vi "Track(topview).vi"() -> ()   [LabVIEW 2014]
uses:
  <vilib>/Utility/file.llb/Write To Spreadsheet File (string).vi
  <vilib>/vision/NI_Vision_Development_Module.lvlib
panel:
  in  "Pause Button":bool
  out "Numeric":dbl
  in  "Start":bool
  in  "Stop Button":bool
  in  "Frame jump":i32=3
  out "Data":dbl[][](array[numeric])
  in  "Grab":bool
  out "Top VIew":cluster{"Numeric":dbl, "Numeric":dbl}[](graph)
  in  "Playback speed":u32(slide)=200
  in  "Progress":i32(slide) step=219843704 scale=-1.0..377.0
  in  "Video path":path
  out "Track":T1(plugin-control)
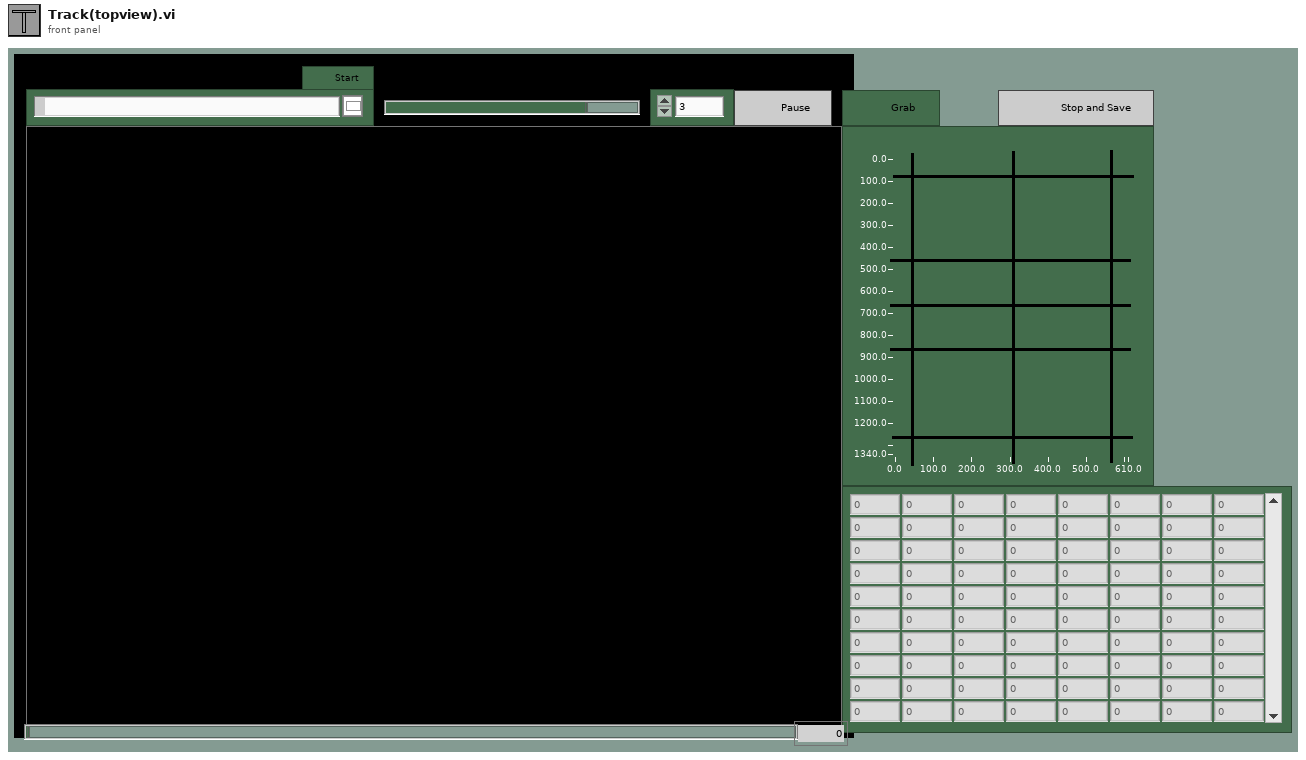
[diagram p1: front panel]
types:
  T1 = typedef "IMAQ Image.ctl" = refnum<image>
  T2 = typedef "Image Type" = u32
  T3 = typedef "AviRefnum.ctl" = refnum<k1>
  T4 = cluster{"width":u32, "height":u32, "framesPerSecond":u32, "compressionFilter":string, "hasData":bool}
  T5 = cluster{cluster{"X":sgl, "Y":sgl}[], cluster{i32, i32}[], "Unit":u32}
  T6 = cluster{"Origin Pixel":cluster{"X":sgl, "Y":sgl}, "Angle Relative to Horizontal (deg)":sgl, "Axis Reference":u32}
  T7 = typedef "Particle Parameters" = i32
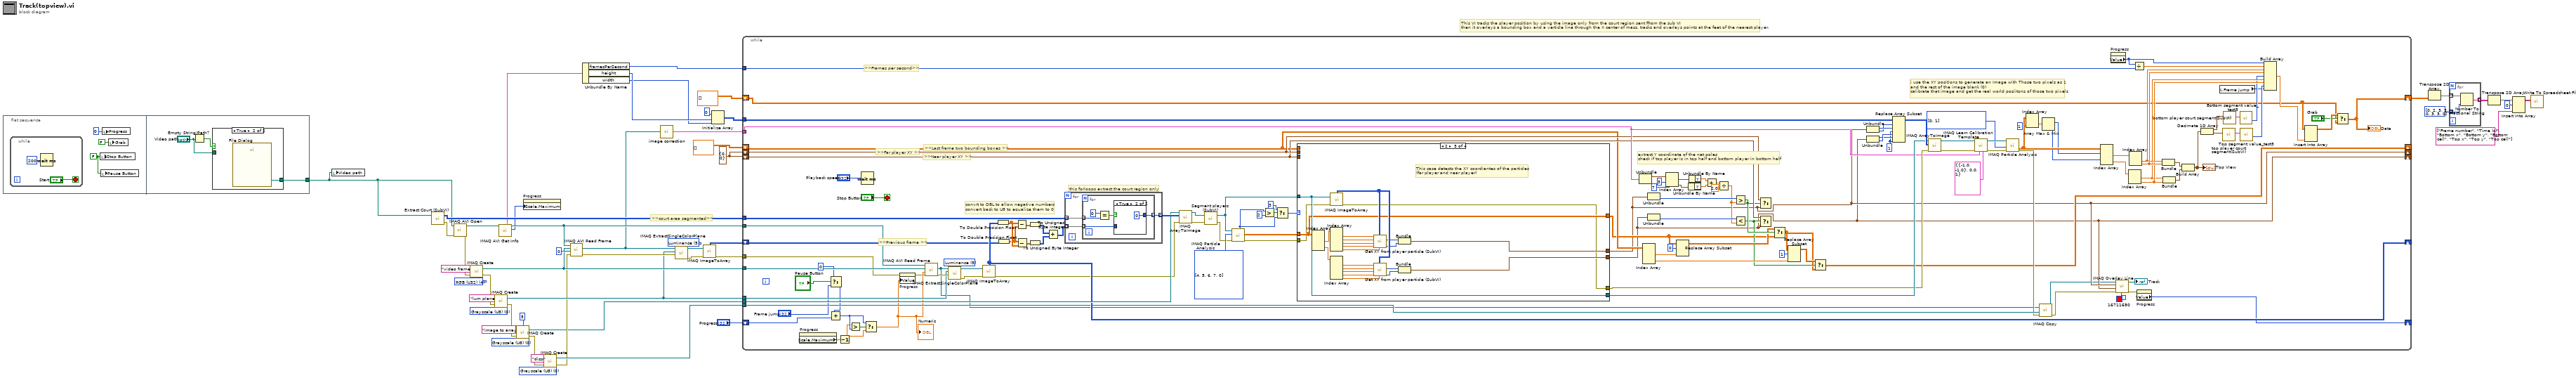
[diagram p0: block diagram]
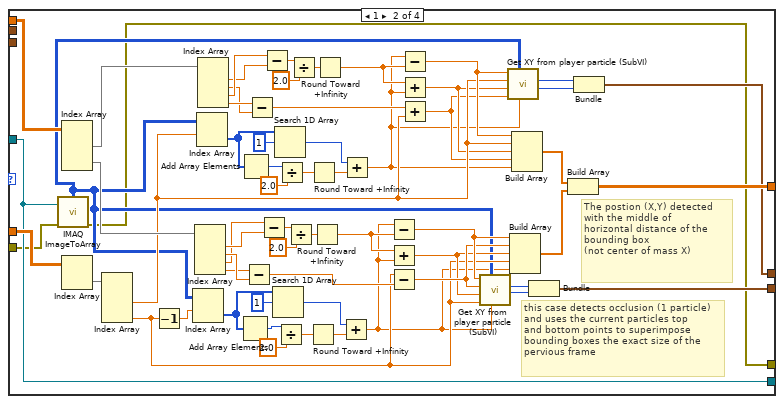
[diagram p4: hidden frame]
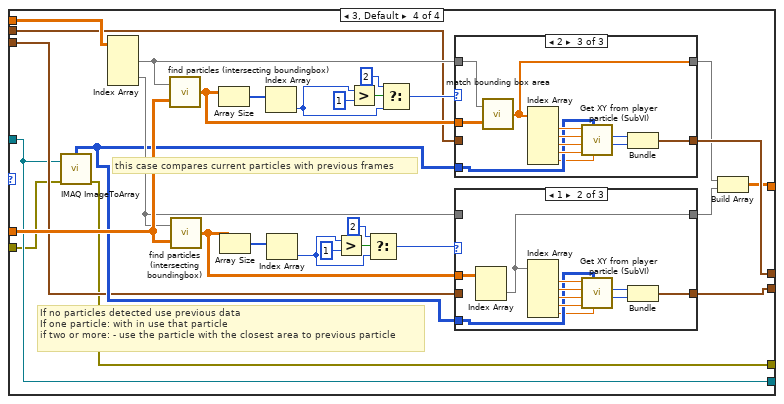
[diagram p5: hidden frame]
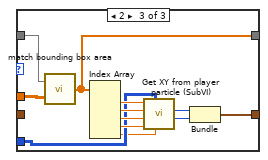
[diagram p7: hidden frame]
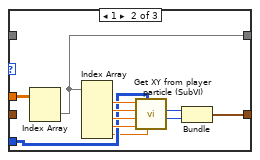
[diagram p9: hidden frame]
diagram:
  w24 = cluster{"X coordinate":i32, "Y coordinate":i32} {"X coordinate"=0, "Y coordinate"=0}
  w37 = T2 0 items=["Grayscale (U8)", "Grayscale (I16)", "Grayscale (SGL)", "Complex (CSG)", "RGB (U32)", "HSL (U32)", "RGB (U64)", "Grayscale (U16)"] ("Image Type")
  w44 = 5 items=["Red", "Green", "Blue", "Hue", "Saturation", "Luminance", "Value", "Intensity"] ("Color Plane")
  w45 = T2 0 items=["Grayscale (U8)", "Grayscale (I16)", "Grayscale (SGL)", "Complex (CSG)", "RGB (U32)", "HSL (U32)", "RGB (U64)", "Grayscale (U16)"] ("Image Type")
  w49 = T2 0 items=["Grayscale (U8)", "Grayscale (I16)", "Grayscale (SGL)", "Complex (CSG)", "RGB (U32)", "HSL (U32)", "RGB (U64)", "Grayscale (U16)"] ("Image Type")
  w47 = T2 4 items=["Grayscale (U8)", "Grayscale (I16)", "Grayscale (SGL)", "Complex (CSG)", "RGB (U32)", "HSL (U32)", "RGB (U64)", "Grayscale (U16)"] ("Image Type")
  # ">>court area segmented>>"
  # "This VI tracks the player position by using the image only from the court region sent ffrom the sub VI\nthen it overlays a bounding box and a verticle line through the X center of mass. tracks and overlays points at the feet of the nearest player."
  n1 = flat-sequence {
    tunnel: [w59] -> w3
    frame #0 {
      w52 = FALSE ("Stop Button")
      n2 = while {
        stop <- "Start" stop-if-true
        n3 = Wait (ms)(milliseconds to wait=u32 200) -> ()  [unwired: 1 out]
      }
      n4 = local write "Stop Button"(w52) -> ()
      n5 = local write "Pause Button"(w52) -> ()
      n6 = local write "Progress"(0 ("Progress")) -> ()
      n7 = local write "Grab"(FALSE ("Grab")) -> ()
    }
    frame #1 {
      n8 = Empty String/Path?(string/path="Video path") -> (empty?=w58:bool)
      n9 = case shown="True" w58 {
        tunnel: [w60 w61] -> w59
        tunnel: "Video path" -> [w60 _]
        frame False {
        }
        frame True {
          n10 = call "File Dialog"() -> ("selected path"=w61:path)  [unwired: 12 in, 3 out]
        }
      }
    }
  }
  n11 = local write "Video path"(w3) -> ()
  n12 = call "Extract Court (SubVI).vi"("AVI Path"=w3) -> ("error out"=w51:errorcluster, "Court pixels out"=w27:u8[][])  [unwired: 1 in]
  n13 = call "IMAQ AVI Open"("error in (no error)"=w51, "AVI Path"=w3) -> ("error out"=w33:errorcluster, "Avi Refnum"=w22:T3)  [unwired: 8 in]
  n14 = call "IMAQ Create"("Image Name"="video frame", "Image Type"=w47, "error in (no error)"=w33) -> ("New Image"=w41:T1, "error out"=w32:errorcluster)  [unwired: 2 in]
  n15 = call "IMAQ Create"("Image Name"="lum plane", "Image Type"=w49, "error in (no error)"=w32) -> ("New Image"=w40:T1, "error out"=w31:errorcluster)  [unwired: 2 in]
  n16 = call "IMAQ AVI Get Info"("Avi Refnum"=w22) -> ("Number of Frames"=w20:u32, "Avi Refnum (duplicate)"=w21:T3, "Frame Data"=w17:T4)  [unwired: 6 in, 2 out]
  n17 = call "IMAQ Create"("Border Size"=5, "Image Name"="image to array", "Image Type"=w45, "error in (no error)"=w31) -> ("New Image"=w26:T1, "error out"=w30:errorcluster)  [unwired: 1 in]
  n18 = property on="Progress" class="Slide (strict)"("Scale.Maximum"=w20) -> ()  [unwired: 2 in, 2 out]
  n19 = call "IMAQ Create"("Image Name"="disp", "Image Type"=w37, "error in (no error)"=w30) -> ("New Image"=w35:T1, "error out"=w29:errorcluster)  [unwired: 2 in]
  n20 = call "IMAQ AVI Read Frame"("error in (no error)"=w29, "Frame Number"=u32 0, "Image"=w41, "Avi Refnum"=w21) -> ("error out"=w43:errorcluster, "Image Out"=w1:T1)  [unwired: 4 in, 2 out]
  n21 = Unbundle By Name(w17) -> ("framesPerSecond"=w12:u32, "height"=w16:u32, "width"=w15:u32)
  n22 = call "image correction.vi"("Image"=w1) -> ("ref points"=w2:T5)
  n23 = call "IMAQ ExtractSingleColorPlane"("Color Plane"=w44, "error in (no error)"=w43, "Image Dst"=w40, "Image Src"=w1) -> ("error out"=w34:errorcluster, "Image Dst Out"=w38:T1)  [unwired: 6 in]
  n24 = call "IMAQ ImageToArray"("error in (no error)"=w34, "Image"=w38) -> ("error out"=w19:errorcluster, "Image Pixels (U8)"=w39:u8[][])  [unwired: 2 in, 3 out]
  n25 = Initialize Array(u8 0 ("element"), w16, w15) -> (w14:u8[][])
  n26 = while {
    tunnel: w21 -> [w155]
    tunnel: w41 -> [w171]
    tunnel: w27 -> [w187]
    tunnel: w40 -> [w172]
    tunnel: w26 -> [w185]
    shift-right: [w184] -> _
    shift-left: w39 -> [w183]
    tunnel: w35 -> [w157]
    shift-right: [w102] -> _
    shift-left: dbl[][] [] ("Particle Measurements (Pixels)") -> [w112]
    shift-right: [w100] -> _
    shift-left: w24 -> [w114]
    shift-right: [w99] -> _
    shift-left: w24 -> [w113]
    shift-right: [w151] -> _
    shift-left: "Progress" -> [w156]
    tunnel: w19 -> [w154]
    tunnel: w14 -> [w150]
    tunnel: w2 -> [w127]
    shift-right: [w128] -> w5
    shift-left: dbl[][] [] -> [w74]
    tunnel: w12 -> [w92]
    stop <- "Stop Button" stop-if-true
    w136 = T7[] [0, 1] items=["Center of Mass X", "Center of Mass Y", "First Pixel X", "First Pixel Y", "Bounding Rect Left", "Bounding Rect Top", "Bounding Rect Right", "Bounding Rect Bottom", "Max Feret Diameter Start X", "Max Feret Diameter Start Y", "Max Feret Diameter End X", "Max Feret Diameter End Y", "Max Horiz. Segment Length Left", "Max Horiz. Segment Length Right", "Max Horiz. Segment Length Row", "-", "Bounding Rect Width", "Bounding Rect Height", "Bounding Rect Diagonal", "Perimeter", "Convex Hull Perimeter", "Holes' Perimeter", "Max Feret Diameter", "Equivalent Ellipse Major Axis", "Equivalent Ellipse Minor Axis", "Equivalent Ellipse Minor Axis (Feret)", "Equivalent Rect Long Side", "Equivalent Rect Short Side", "Equivalent Rect Diagonal", "Equivalent Rect Short Side (Feret)", "Average Horiz. Segment Length", "Average Vert. Segment Length", "Hydraulic Radius", "Waddel Disk Diameter", "-", "Area", "Holes' Area", "Particle & Holes' Area", "Convex Hull Area", "Image Area", "-", "Number of Holes", "Number of Horiz. Segments", "Number of Vert. Segments", "-", "Orientation", "Max Feret Diameter Orientation", "-", "% Area/Image Area", "% Area/(Particle & Holes' Area)", "Ratio of Equivalent Ellipse Axes", "Ratio of Equivalent Rect Sides", "-", "Elongation Factor", "Compactness Factor", "Heywood Circularity Factor", "Type Factor", "-", "Sum X", "Sum Y", "Sum XX", "Sum XY", "Sum YY", "Sum XXX", "Sum XXY", "Sum XYY", "Sum YYY", "-", "Moment of Inertia XX", "Moment of Inertia XY", "Moment of Inertia YY", "Moment of Inertia XXX", "Moment of Inertia XXY", "Moment of Inertia XYY", "Moment of Inertia YYY", "Norm. Moment of Inertia XX", "Norm. Moment of Inertia XY", "Norm. Moment of Inertia YY", "Norm. Moment of Inertia XXX", "Norm. Moment of Inertia XXY", "Norm. Moment of Inertia XYY", "Norm. Moment of Inertia YYY", "Hu Moment 1", "Hu Moment 2", "Hu Moment 3", "Hu Moment 4", "Hu Moment 5", "Hu Moment 6", "Hu Moment 7"] ("Real-World Measurements")
    w145 = u8 1 ("new element/subarray")
    w173 = T7[] [4, 5, 6, 7, 0] items=["Center of Mass X", "Center of Mass Y", "First Pixel X", "First Pixel Y", "Bounding Rect Left", "Bounding Rect Top", "Bounding Rect Right", "Bounding Rect Bottom", "Max Feret Diameter Start X", "Max Feret Diameter Start Y", "Max Feret Diameter End X", "Max Feret Diameter End Y", "Max Horiz. Segment Length Left", "Max Horiz. Segment Length Right", "Max Horiz. Segment Length Row", "-", "Bounding Rect Width", "Bounding Rect Height", "Bounding Rect Diagonal", "Perimeter", "Convex Hull Perimeter", "Holes' Perimeter", "Max Feret Diameter", "Equivalent Ellipse Major Axis", "Equivalent Ellipse Minor Axis", "Equivalent Ellipse Minor Axis (Feret)", "Equivalent Rect Long Side", "Equivalent Rect Short Side", "Equivalent Rect Diagonal", "Equivalent Rect Short Side (Feret)", "Average Horiz. Segment Length", "Average Vert. Segment Length", "Hydraulic Radius", "Waddel Disk Diameter", "-", "Area", "Holes' Area", "Particle & Holes' Area", "Convex Hull Area", "Image Area", "-", "Number of Holes", "Number of Horiz. Segments", "Number of Vert. Segments", "-", "Orientation", "Max Feret Diameter Orientation", "-", "% Area/Image Area", "% Area/(Particle & Holes' Area)", "Ratio of Equivalent Ellipse Axes", "Ratio of Equivalent Rect Sides", "-", "Elongation Factor", "Compactness Factor", "Heywood Circularity Factor", "Type Factor", "-", "Sum X", "Sum Y", "Sum XX", "Sum XY", "Sum YY", "Sum XXX", "Sum XXY", "Sum XYY", "Sum YYY", "-", "Moment of Inertia XX", "Moment of Inertia XY", "Moment of Inertia YY", "Moment of Inertia XXX", "Moment of Inertia XXY", "Moment of Inertia XYY", "Moment of Inertia YYY", "Norm. Moment of Inertia XX", "Norm. Moment of Inertia XY", "Norm. Moment of Inertia YY", "Norm. Moment of Inertia XXX", "Norm. Moment of Inertia XXY", "Norm. Moment of Inertia XYY", "Norm. Moment of Inertia YYY", "Hu Moment 1", "Hu Moment 2", "Hu Moment 3", "Hu Moment 4", "Hu Moment 5", "Hu Moment 6", "Hu Moment 7"] ("Pixel Measurements")
    w188 = 5 items=["Red", "Green", "Blue", "Hue", "Saturation", "Luminance", "Value", "Intensity"] ("Color Plane")
    # ">>Frames per second>>"
    # "extract Y coordinate of the net poles\ncheck if top player is in top half and bottom player in bottom half"
    # "i use the XY positions to generate an Image with Those two pixels as 1 \nand the rest of the image blank (0)\ncalibrate that image and get the real world posiitons of those two pixels"
    # ">>Last frame two bounding boxes >>"
    # ">>Far player XY >>"
    # ">>Near player XY >>"
    # ">>Previous frame >>"
    # "convrt to DBL to allow negative numbers\nconvert back to U8 to equalize them to 0"
    # "this forloops extract the court region only"
    n27 = property on="Progress" class="Slide (strict)"() -> ("Scale.Maximum"=w72:dbl)  [unwired: 2 in, 2 out]
    n28 = Select(t=0, s="Pause Button", f="Frame jump") -> (s? t:f=w64:i32)
    n29 = Add(x=w64, y=w156) -> (x+y=w70:i32)
    n30 = Decrement(x=w72) -> (x-1=w69:dbl)
    n31 = Greater?(x=w69, y=w70) -> (0:w71:bool)
    n32 = Wait (ms)(milliseconds to wait="Playback speed") -> ()  [unwired: 1 out]
    n33 = Select(t=w70, s=w71, f=w69) -> (s? t:f=w62:dbl)
    "Numeric" <- w62
    n34 = property on="Progress" class="Slide (strict)"(error in=w154, "Value"=w62) -> (error out=w153:errorcluster)  [unwired: 1 in, 1 out]
    n35 = call "IMAQ AVI Read Frame"("error in (no error)"=w153, "Frame Number"=w62, "Image"=w171, "Avi Refnum"=w155) -> ("error out"=w189:errorcluster, "Image Out"=w90:T1)  [unwired: 4 in, 2 out]
    n36 = call "IMAQ ExtractSingleColorPlane"("Color Plane"=w188, "error in (no error)"=w189, "Image Dst"=w172, "Image Src"=w90) -> ("error out"=w175:errorcluster, "Image Dst Out"=w89:T1)  [unwired: 6 in]
    n37 = call "IMAQ ImageToArray"("error in (no error)"=w175, "Image"=w89) -> ("error out"=w174:errorcluster, "Image Pixels (U8)"=w184:u8[][])  [unwired: 2 in, 3 out]
    n38 = To Double Precision Float(number=w184) -> (double precision float=w179:dbl[][])
    n39 = To Double Precision Float(number=w183) -> (double precision float=w178:dbl[][])
    n40 = Subtract(x=w179, y=w178) -> (x-y=w177:dbl[][])
    n41 = Subtract(x=w178, y=w179) -> (x-y=w176:dbl[][])
    n42 = To Unsigned Byte Integer(number=w177) -> (unsigned 8bit integer=w182:u8[][])
    n43 = To Unsigned Byte Integer(number=w176) -> (unsigned 8bit integer=w181:u8[][])
    n44 = Add(x=w182, y=w181) -> (x+y=w180:u8[][])
    n45 = for {
      tunnel: w187 -> [w360] mode=indexing
      tunnel: [w359] -> w186 mode=indexing
      tunnel: w180 -> [w358] mode=indexing
      n46 = for {
        tunnel: w360 -> [w365] mode=indexing
        tunnel: [w362] -> w359 mode=indexing
        tunnel: w358 -> [w361] mode=indexing
        n47 = Equal?(x=u8 0, y=w365) -> (x = y?=w363:bool)
        n48 = case shown="True" w363 {
          tunnel: [w366 u8 0 ("x")] -> w362
          tunnel: w361 -> [w366 _]
          frame False {
          }
          frame True {
          }
        }
      }
    }
    n49 = call "IMAQ ArrayToImage"("error in (no error)"=w174, "Image Pixels (U8)"=w186, "Image"=w185) -> ("error out"=w169:errorcluster, "Image Out"=w170:T1)  [unwired: 7 in]
    n50 = call "Segment players (SubVI).vi"("error In"=w169, "Image In"=w170) -> ("error out"=w163:errorcluster, "Image Out"=w161:T1)
    n51 = call "IMAQ Particle Analysis"("error in (no error)"=w163, "Pixel Measurements"=w173, "Image"=w161) -> ("error out"=w162:errorcluster, "Particle Measurements (Pixels)"=w160:dbl[][], "Number of Particles"=w165:i32)  [unwired: 3 in, 3 out]
    n52 = Greater?(x=w165, y=2) -> (0:w168:bool)
    n53 = Select(t=3 ("y"), s=w168, f=w165) -> (s? t:f=w164:i32)
    n54 = case shown="2" w164 {
      tunnel: [w193 w220 w274 w284] -> w143
      tunnel: w160 -> [_ w255 w262 w304]
      tunnel: w162 -> [w190 w196 w259 w280]
      tunnel: w161 -> [w193 w220 w274 w284]
      tunnel: [w191 w204 w264 w286] -> w99
      tunnel: [w192 w211 w263 w285] -> w100
      tunnel: [w194 w221 w262 w281] -> w101
      tunnel: w112 -> [w194 w245 _ w307]
      tunnel: w114 -> [w192 _ _ w292]
      tunnel: w113 -> [w191 _ _ w287]
      tunnel: [w190 w195 w258 w279] -> w142
      frame 0 {
        # "This case identifies frames where no particles are detected and keeps the same values from the\nprevious frame"
      }
      frame 1 {
        # "The postion (X,Y) detected with the middle of \nhorizontal distance of the bounding box\n(not center of mass X)"
        # "this case detects occlusion (1 particle)\nand uses the current particles top \nand bottom points to superimpose \nbounding boxes the exact size of the \npervious frame"
        n55 = call "IMAQ ImageToArray"("error in (no error)"=w196, "Image"=w220) -> ("error out"=w195:errorcluster, "Image Pixels (U8)"=w203:u8[][])  [unwired: 2 in, 3 out]
        n56 = Index Array(array=w245) -> (element #1=w253:dbl[], element #2=w225:dbl[])  [unwired: 4 in]
        n57 = Index Array(array=w255) -> (element=w254:dbl[])  [unwired: 2 in]
        n58 = Index Array(array=w254) -> (element #2=w216:dbl, element #4=w207:dbl)  [unwired: 4 in, 2 out]
        n59 = Decrement(x=w207) -> (x-1=w218:dbl)
        n60 = Index Array(array=w203, index (row)=w218) -> (element=w240:u8[])  [unwired: 1 in]
        n61 = Index Array(array=w225) -> (element #1=w229:dbl, element #2=w232:dbl, element #3=w228:dbl, element #4=w231:dbl)  [unwired: 4 in]
        n62 = Index Array(array=w203, index (row)=w216) -> (element=w233:u8[])  [unwired: 1 in]
        n63 = Index Array(array=w253) -> (element #1=w249:dbl, element #2=w246:dbl, element #3=w250:dbl, element #4=w247:dbl)  [unwired: 4 in]
        n64 = Add Array Elements(numeric array=w240) -> (sum=w241:u8)
        n65 = Add Array Elements(numeric array=w233) -> (sum=w237:u8)
        n66 = Subtract(x=w231, y=w232) -> (x-y=w219:dbl)
        n67 = Subtract(x=w247, y=w246) -> (x-y=w224:dbl)
        n68 = Subtract(x=w228, y=w229) -> (x-y=w227:dbl)
        n69 = Subtract(x=w250, y=w249) -> (x-y=w251:dbl)
        n70 = Search 1D Array(1D array=w240, element=u8 1) -> (index of element=w239:i32)  [unwired: 1 in]
        n71 = Search 1D Array(1D array=w233, element=u8 1) -> (index of element=w238:i32)  [unwired: 1 in]
        n72 = Divide(x=w241, y=2.0) -> (x/y=w242:dbl)
        n73 = Divide(x=w237, y=2.0) -> (x/y=w236:dbl)
        n74 = Divide(x=w227, y=2.0) -> (x/y=w230:dbl)
        n75 = Divide(x=w251, y=2.0) -> (x/y=w248:dbl)
        n76 = Round Toward +Infinity(x=w242) -> (ceil(x): smallest int >= x=w201:dbl)
        n77 = Round Toward +Infinity(x=w236) -> (ceil(x): smallest int >= x=w200:dbl)
        n78 = Round Toward +Infinity(x=w230) -> (ceil(x): smallest int >= x=w202:dbl)
        n79 = Round Toward +Infinity(x=w248) -> (ceil(x): smallest int >= x=w199:dbl)
        n80 = Add(x=w239, y=w201) -> (x+y=w197:dbl)
        n81 = Add(x=w238, y=w200) -> (x+y=w198:dbl)
        n82 = Subtract(x=w197, y=w202) -> (x-y=w210:dbl)
        n83 = Add(x=w202, y=w197) -> (x+y=w208:dbl)
        n84 = Subtract(x=w207, y=w219) -> (x-y=w209:dbl)
        n85 = Subtract(x=w198, y=w199) -> (x-y=w217:dbl)
        n86 = Add(x=w199, y=w198) -> (x+y=w215:dbl)
        n87 = Add(x=w224, y=w216) -> (x+y=w214:dbl)
        n88 = call "Get XY from player particle (SubVI).vi"("Center of mass X"=w197, "Image in Pixels (U8)"=w203, "Particle bounding rect bottom"=w207, "Particle bounding rect right"=w208, "Particle bounding rect top"=w209, "Particle bounding rect left"=w210) -> ("Y coordinate"=w205:i32, "X coordinate"=w206:i32)  [unwired: 1 in, 1 out]
        n89 = call "Get XY from player particle (SubVI).vi"("Center of mass X"=w198, "Image in Pixels (U8)"=w203, "Particle bounding rect bottom"=w214, "Particle bounding rect right"=w215, "Particle bounding rect top"=w216, "Particle bounding rect left"=w217) -> ("Y coordinate"=w212:i32, "X coordinate"=w213:i32)  [unwired: 1 in, 1 out]
        n90 = Build Array(w210, w209, w208, w207, w197) -> (w222:dbl[])
        n91 = Build Array(w217, w216, w215, w214, w198) -> (w223:dbl[])
        n92 = Bundle("X coordinate"=w206, "Y coordinate"=w205) -> (w204:cluster{"X coordinate":i32, "Y coordinate":i32})  [unwired: 1 in]
        n93 = Build Array(w223, w222) -> (w221:dbl[][])
        n94 = Bundle("X coordinate"=w213, "Y coordinate"=w212) -> (w211:cluster{"X coordinate":i32, "Y coordinate":i32})  [unwired: 1 in]
      }
      frame 2 {
        # "This case detects the XY coordiantes of the particles\n(far player and near player)"
        n95 = Index Array(array=w262) -> (element #1=w268:dbl[], element #2=w267:dbl[])  [unwired: 4 in]
        n96 = call "IMAQ ImageToArray"("error in (no error)"=w259, "Image"=w274) -> ("error out"=w258:errorcluster, "Image Pixels (U8)"=w269:u8[][])  [unwired: 2 in, 3 out]
        n97 = Index Array(array=w268) -> (element #1=w278:dbl, element #2=w277:dbl, element #3=w276:dbl, element #4=w275:dbl, element #5=w261:dbl)  [unwired: 5 in]
        n98 = Index Array(array=w267) -> (element #1=w270:dbl, element #2=w271:dbl, element #3=w272:dbl, element #4=w273:dbl, element #5=w260:dbl)  [unwired: 5 in]
        n99 = call "Get XY from player particle (SubVI).vi"("Center of mass X"=w261, "Image in Pixels (U8)"=w269, "Particle bounding rect bottom"=w275, "Particle bounding rect right"=w276, "Particle bounding rect top"=w277, "Particle bounding rect left"=w278) -> ("Y COM"=w257:i32, "X coordinate"=w266:i32)  [unwired: 1 in, 1 out]
        n100 = call "Get XY from player particle (SubVI).vi"("Center of mass X"=w260, "Image in Pixels (U8)"=w269, "Particle bounding rect bottom"=w273, "Particle bounding rect right"=w272, "Particle bounding rect top"=w271, "Particle bounding rect left"=w270) -> ("Y COM"=w256:i32, "X coordinate"=w265:i32)  [unwired: 1 in, 1 out]
        n101 = Bundle("X coordinate"=w266, "Y COM"=w257) -> (w263:cluster{"X coordinate":i32, "Y COM":i32})  [unwired: 1 in]
        n102 = Bundle("X coordinate"=w265, "Y COM"=w256) -> (w264:cluster{"X coordinate":i32, "Y COM":i32})  [unwired: 1 in]
      }
      frame 3, Default {
        # "If no particles detected use previous data\nIf one particle: with in use that particle\nif two or more: - use the particle with the closest area to previous particle"
        # "this case compares current particles with previous frames"
        n103 = call "IMAQ ImageToArray"("error in (no error)"=w280, "Image"=w284) -> ("error out"=w279:errorcluster, "Image Pixels (U8)"=w288:u8[][])  [unwired: 2 in, 3 out]
        n104 = Index Array(array=w307) -> (element #1=w303:dbl[], element #2=w291:dbl[])  [unwired: 4 in]
        n105 = call "find particles (intersecting boundingbox).vi"("Particle Measurements in (bounding boxes)"=w304, "bounding box in"=w303) -> ("Particles within bounding box"=w302:dbl[][])
        n106 = call "find particles (intersecting boundingbox).vi"("Particle Measurements in (bounding boxes)"=w304, "bounding box in"=w291) -> ("Particles within bounding box"=w289:dbl[][])
        n107 = Array Size(array=w302) -> (size(s)=w306:i32[])
        n108 = Array Size(array=w289) -> (size(s)=w305:i32[])
        n109 = Index Array(array=w306) -> (element=w294:i32)  [unwired: 1 in]
        n110 = Index Array(array=w305) -> (element=w295:i32)  [unwired: 1 in]
        n111 = Greater?(x=w295, y=1) -> (0:w298:bool)
        n112 = Greater?(x=w294, y=1) -> (0:w299:bool)
        n113 = Select(t=2 ("y"), s=w298, f=w295) -> (s? t:f=w290:i32)
        n114 = Select(t=2 ("y"), s=w299, f=w294) -> (s? t:f=w293:i32)
        n115 = case shown="2" w293 {
          tunnel: w303 -> [w334 _ w349]
          tunnel: w302 -> [_ w345 w348]
          tunnel: [w334 w336 w347] -> w283
          tunnel: w288 -> [_ w338 w351]
          tunnel: [w333 w337 w350] -> w285
          tunnel: w292 -> [w333 _ _]
          frame 0, Default {
          }
          frame 1 {
            n116 = Index Array(array=w345) -> (element=w336:dbl[])  [unwired: 2 in]
            n117 = Index Array(array=w336) -> (element #1=w342:dbl, element #2=w341:dbl, element #3=w340:dbl, element #4=w339:dbl, element #5=w335:dbl)  [unwired: 5 in]
            n118 = call "Get XY from player particle (SubVI).vi"("Center of mass X"=w335, "Image in Pixels (U8)"=w338, "Particle bounding rect bottom"=w339, "Particle bounding rect right"=w340, "Particle bounding rect top"=w341, "Particle bounding rect left"=w342) -> ("Y coordinate"=w343:i32, "X coordinate"=w344:i32)  [unwired: 1 in, 1 out]
            n119 = Bundle("X coordinate"=w344, "Y coordinate"=w343) -> (w337:cluster{"X coordinate":i32, "Y coordinate":i32})  [unwired: 1 in]
          }
          frame 2 {
            n120 = call "match bounding box area.vi"("particle measurements (bounding box)"=w348, "bounding box in"=w349) -> ("matching bounding box"=w347:dbl[])
            n121 = Index Array(array=w347) -> (element #1=w355:dbl, element #2=w354:dbl, element #3=w353:dbl, element #4=w352:dbl, element #5=w346:dbl)  [unwired: 5 in]
            n122 = call "Get XY from player particle (SubVI).vi"("Center of mass X"=w346, "Image in Pixels (U8)"=w351, "Particle bounding rect bottom"=w352, "Particle bounding rect right"=w353, "Particle bounding rect top"=w354, "Particle bounding rect left"=w355) -> ("Y coordinate"=w356:i32, "X coordinate"=w357:i32)  [unwired: 1 in, 1 out]
            n123 = Bundle("X coordinate"=w357, "Y coordinate"=w356) -> (w350:cluster{"X coordinate":i32, "Y coordinate":i32})  [unwired: 1 in]
          }
        }
        n124 = case shown="1" w290 {
          tunnel: w291 -> [w309 _ w324]
          tunnel: w289 -> [_ w320 w323]
          tunnel: [w309 w311 w322] -> w282
          tunnel: w288 -> [_ w313 w326]
          tunnel: [w308 w312 w325] -> w286
          tunnel: w287 -> [w308 _ _]
          frame 0, Default {
          }
          frame 1 {
            n125 = Index Array(array=w320) -> (element=w311:dbl[])  [unwired: 2 in]
            n126 = Index Array(array=w311) -> (element #1=w317:dbl, element #2=w316:dbl, element #3=w315:dbl, element #4=w314:dbl, element #5=w310:dbl)  [unwired: 5 in]
            n127 = call "Get XY from player particle (SubVI).vi"("Center of mass X"=w310, "Image in Pixels (U8)"=w313, "Particle bounding rect bottom"=w314, "Particle bounding rect right"=w315, "Particle bounding rect top"=w316, "Particle bounding rect left"=w317) -> ("Y coordinate"=w318:i32, "X coordinate"=w319:i32)  [unwired: 1 in, 1 out]
            n128 = Bundle("X coordinate"=w319, "Y coordinate"=w318) -> (w312:cluster{"X coordinate":i32, "Y coordinate":i32})  [unwired: 1 in]
          }
          frame 2 {
            n129 = call "match bounding box area.vi"("particle measurements (bounding box)"=w323, "bounding box in"=w324) -> ("matching bounding box"=w322:dbl[])
            n130 = Index Array(array=w322) -> (element #1=w330:dbl, element #2=w329:dbl, element #3=w328:dbl, element #4=w327:dbl, element #5=w321:dbl)  [unwired: 5 in]
            n131 = call "Get XY from player particle (SubVI).vi"("Center of mass X"=w321, "Image in Pixels (U8)"=w326, "Particle bounding rect bottom"=w327, "Particle bounding rect right"=w328, "Particle bounding rect top"=w329, "Particle bounding rect left"=w330) -> ("Y coordinate"=w331:i32, "X coordinate"=w332:i32)  [unwired: 1 in, 1 out]
            n132 = Bundle("X coordinate"=w332, "Y coordinate"=w331) -> (w325:cluster{"X coordinate":i32, "Y coordinate":i32})  [unwired: 1 in]
          }
        }
        n133 = Build Array(w283, w282) -> (w281:dbl[][])
      }
    }
    n134 = Unbundle(w127) -> (w126:cluster{"X":sgl, "Y":sgl}[])  [unwired: 2 out]
    n135 = Index Array(array=w112) -> (element #1=w110:dbl[], element #2=w106:dbl[])  [unwired: 4 in]
    n136 = Unbundle(w99) -> ("Y coordinate"=w116:i32)  [unwired: 1 out]
    n137 = Unbundle(w100) -> ("Y coordinate"=w117:i32)  [unwired: 1 out]
    n138 = Index Array(array=w126, index #1=3 ("index"), index #2=7 ("index")) -> (element #1=w123:cluster{"X":sgl, "Y":sgl}, element #2=w122:cluster{"X":sgl, "Y":sgl})
    n139 = Replace Array Subset(array=w101, new element=w110, index (row)=0) -> (w109:dbl[][])  [unwired: 1 in]
    n140 = Unbundle By Name(w122) -> ("Y"=w120:sgl)
    n141 = Unbundle By Name(w123) -> ("Y"=w121:sgl)
    n142 = Add(x=w121, y=w120) -> (x+y=w119:sgl)
    n143 = Divide(x=w119, y=sgl 2.0) -> (x/y=w115:sgl)
    n144 = Greater?(x=w117, y=w115) -> (0:w111:bool)
    n145 = Less?(x=w116, y=w115) -> (x < y?=w104:bool)
    n146 = Select(t=w114, s=w111, f=w100) -> ()  [unwired: 1 out]
    n147 = Select(t=w113, s=w104, f=w99) -> ()  [unwired: 1 out]
    n148 = Select(t=w109, s=w111, f=w101) -> (s? t:f=w103:dbl[][])
    n149 = Replace Array Subset(array=w103, new element=w106, index (row)=1) -> (w105:dbl[][])  [unwired: 1 in]
    n150 = Select(t=w105, s=w104, f=w103) -> (s? t:f=w102:dbl[][])
    n151 = Unbundle(w99) -> ("X coordinate"=w146:i32, "Y coordinate"=w147:i32)
    n152 = Unbundle(w100) -> ("X coordinate"=w149:i32, "Y coordinate"=w148:i32)
    n153 = Replace Array Subset(array=w150, new element #1=w145, index (row) #1=w148, index (col) #1=w149, new element #2=w145, index (row) #2=w147, index (col) #2=w146) -> (w144:u8[][])
    n154 = call "IMAQ ArrayToImage"("error in (no error)"=w142, "Image Pixels (U8)"=w144, "Image"=w143) -> ("error out"=w139:errorcluster, "Image Out"=w140:T1)  [unwired: 7 in]
    n155 = call "IMAQ Learn Calibration Template"("Calibration Axis Info"=T6 {"Origin Pixel"={"X"=-1.0, "Y"=-1.0}, "Angle Relative to Horizontal (deg)"=0.0, "Axis Reference"=1}, "Reference Points"=w127, "error in (no error)"=w139, "Image"=w140) -> ("error out"=w138:errorcluster, "Calibrated Image"=w137:T1)  [unwired: 5 in, 1 out]
    n156 = call "IMAQ Particle Analysis"("error in (no error)"=w138, "Real-World Measurements"=w136, "Image"=w137) -> ("error out"=w135:errorcluster, "Particle Measurements (Real-World)"=w85:dbl[][])  [unwired: 3 in, 4 out]
    n157 = Index Array(array=w85, index (col)=1 ("disabled index (col)")) -> (element=w83:dbl[])  [unwired: 1 in]
    n158 = call "IMAQ Copy"("error in (no error)"=w135, "Image Dst"=w157, "Image Src"=w90) -> ("error out"=w97:errorcluster, "Image Dst Out"=w98:T1)  [unwired: 3 in]
    n159 = Array Max & Min(array=w83) -> (max index (indices)=w82:i32, min index (indices)=w81:i32)  [unwired: 2 out]
    n160 = Index Array(array=w85, index (row) #1=w82, index (row) #2=w81) -> (element #1=w134:dbl[], element #2=w133:dbl[])  [unwired: 2 in]
    n161 = property on="Progress" class="Slide (strict)"() -> ("Value"=w93:i32)  [unwired: 2 in, 2 out]
    n162 = call "IMAQ Overlay Line"("Color"=u32 16711680, "error in (no error)"=w97, "End Point"=w99, "Start Point"=w100, "Image"=w98) -> ("error out"=w152:errorcluster, "Image Out"=→"Track":T1)  [unwired: 5 in]
    n163 = Index Array(array=w133) -> (element #1=w76:dbl, element #2=w77:dbl)  [unwired: 2 in]
    n164 = Index Array(array=w134) -> (element #1=w96:dbl, element #2=w95:dbl)  [unwired: 2 in]
    n165 = Divide(x=w93, y=w92) -> (x/y=w91:dbl)
    n166 = property on="Progress" class="Slide (strict)"(error in=w152) -> ("Value"=w151:i32)  [unwired: 1 in, 2 out]
    n167 = Bundle("Numeric"=w96, "Numeric"=w95) -> (w130:cluster{"Numeric":dbl, "Numeric":dbl})  [unwired: 1 in]
    n168 = Bundle("Numeric"=w76, "Numeric"=w77) -> (w129:cluster{"Numeric":dbl, "Numeric":dbl})  [unwired: 1 in]
    n169 = Build Array(w130, w129) -> (w88:cluster{"Numeric":dbl, "Numeric":dbl}[])
    "Top VIew" <- w88
    n170 = Decimate 1D Array(w88) -> (w80:cluster{"Numeric":dbl, "Numeric":dbl}[], w79:cluster{"Numeric":dbl, "Numeric":dbl}[])
    n171 = local read "Frame jump"() -> (w68:i32)
    n172 = call "top player court segment(SubVI).vi"("Top player position"=w79) -> ("Top player segment position"=w87:string)  [unwired: 10 in]
    n173 = call "bottom player court segment(SubVI).vi"("Bottom player position"=w80) -> ("Bottom player segment position"=w86:string)  [unwired: 10 in]
    n174 = call "Bottom segment value_test3.vi"("Bottom player segment position"=w86) -> ("Bottom player segment"=w75:i32)  [unwired: 9 in, 1 out]
    n175 = call "Top segment value_test3.vi"("Top player segment position"=w87) -> ("Top player segment value"=w78:i32)  [unwired: 9 in, 1 out]
    n176 = Build Array(w93, w91, w96, w95, w75, w76, w77, w78, w68) -> (w94:dbl[])
    n177 = Insert Into Array(array=w74, new element=w94) -> (w132:dbl[][])  [unwired: 2 in]
    n178 = Select(t=w132, s="Grab", f=w74) -> (s? t:f=w128:dbl[][])
    "Data" <- w128
  }
  n179 = Transpose 2D Array(2D array=w5) -> (transposed array=w8:dbl[][])
  n180 = for {
    tunnel: w8 -> [w370] mode=indexing
    tunnel: i16[] [0, 2, 3, 3, 0, 3, 3, 0] -> [w369] mode=indexing
    tunnel: [w368] -> w6 mode=indexing
    n181 = Number To Fractional String(number=w370, precision (6)=w369) -> (F-format string=w368:string[])  [unwired: 2 in]
  }
  n182 = Transpose 2D Array(2D array=w6) -> (transposed array=w4:string[][])
  n183 = Insert Into Array(array=w4, index (row)=0, new element=string[] ["Frame number", "Time (s)", "Bottom x", "Bottom y", "Bottom cell", "Top x", "Top y", "Top cell"] ("new element/subarray")) -> (w9:string[][])  [unwired: 1 in]
  n184 = call-poly <vilib>:"Write To Spreadsheet File.vi"("2D data"=w9) -> ()  [unwired: 7 in, 1 out]
